vi "游标-删除所有.vi"(5 "reference in":refnum<vi>) -> (2 "reference out":refnum<vi>)   [LabVIEW 2013]
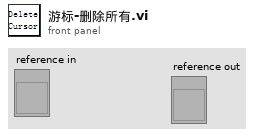
[diagram p1: front panel]
types:
  T1 = typedef "LVCursorListTypeDef.ctl" = cluster{"Name":string, "Color":u32, "Style":u8, "Point Style":u8, "Name Visible":bool, "Allow Drag":bool, "Cursor Mode":u32, "Plot":i32, "Index":i32, "Position":cluster{"X":dbl, "Y":dbl}, "X Scale":u32, "Y Scale":u32, "Watch Plots":i32[], "Watch All Plots":bool, "Plot Area":i32, "Label Offset":cluster{"X":dbl, "Y":dbl}}[]
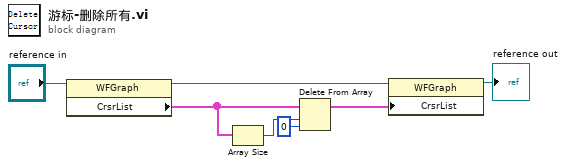
[diagram p0: block diagram]
diagram:
  n1 = property class="WFGraph"(reference="reference in") -> (reference out=w3:refnum<vi>, "CrsrList"=w2:T1)  [unwired: 1 in, 1 out]
  n2 = Array Size(array=w2) -> (size(s)=w7:i32)
  n3 = Delete From Array(array=w2, length=w7, index=0) -> (array with subset deleted=w5:T1)  [unwired: 1 out]
  n4 = property class="WFGraph"(reference=w3, "CrsrList"=w5) -> (reference out=→"reference out":refnum<vi>)  [unwired: 1 in, 1 out]
